vi "Write Boolean.vi"(8 "error in (no error)":errorcluster, 10 "Boolean":bool, 11 "Boolean in":refnum<class "Boolean.lvclass">) -> (0 "error out":errorcluster, 3 "Boolean out":refnum<class "Boolean.lvclass">)   [LabVIEW 2013, in "HardwareCharacterization.lvlib" / "Boolean.lvclass"]
uses:
  Boolean.lvclass
  Boolean.lvclass/Boolean.ctl
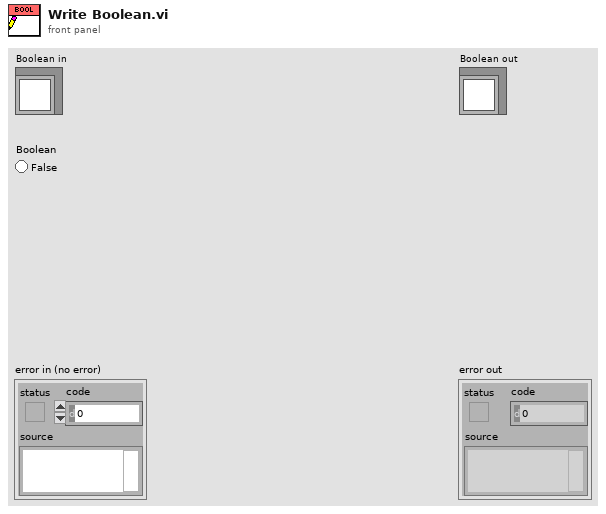
[diagram p1: front panel]
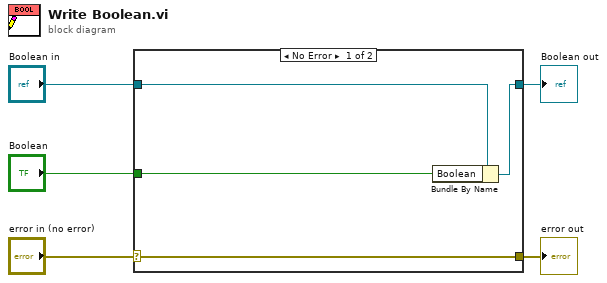
[diagram p0: block diagram]
diagram:
  n1 = case shown="No Error" "error in (no error)" {
    selector: "error in (no error)" -> [w9 w10]
    tunnel: [w9 w10] -> w4
    tunnel: [w7 w11] -> w2
    tunnel: "Boolean in" -> [w8 w11]
    tunnel: "Boolean" -> [w6 _]
    frame No Error {
      n2 = Bundle By Name(cluster=w8, "Boolean"=w6) -> (w7:refnum<class "Boolean.lvclass">)
    }
    frame Error {
    }
  }
  "error out" <- w4
  "Boolean out" <- w2
